vi "uTTA_ucf_WriteChannelCal.vi"(4 "LinGain":dbl, 5 "QuadGain":dbl, 6 "Offset":dbl, 7 "Section":string, 8 "error in (no error)":errorcluster, 9 "Cal Status":T1, 11 "ucf FileRef in":T2) -> (0 "error out":errorcluster, 3 "ucf FileRef out":T2)   [LabVIEW 2021]
uses:
  <vilib>/Utility/config.llb/Config Data RefNum.ctl
  uTTA_Device_Driver/uTTA_Controls/CTL_uTTA_TSP_CalStatus.ctl
  <vilib>/Utility/config.llb/Write Key (U32).vi
  <vilib>/Utility/config.llb/NI_LVConfig.lvlib
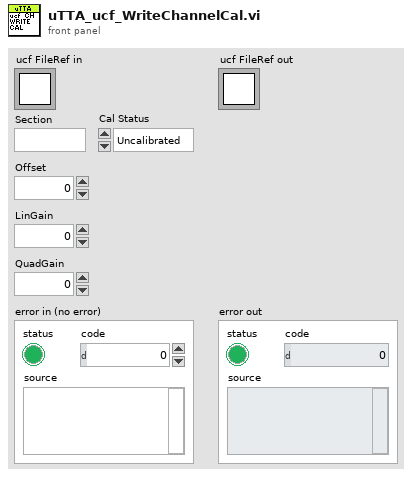
[diagram p1: front panel]
types:
  T1 = typedef "CTL_uTTA_TSP_CalStatus.ctl" = enum16{"Uncalibrated", "Calibrated", "Dummy"}
  T2 = typedef "NI_LVConfig.lvlib/Config Data RefNum.ctl" = refnum<k1>
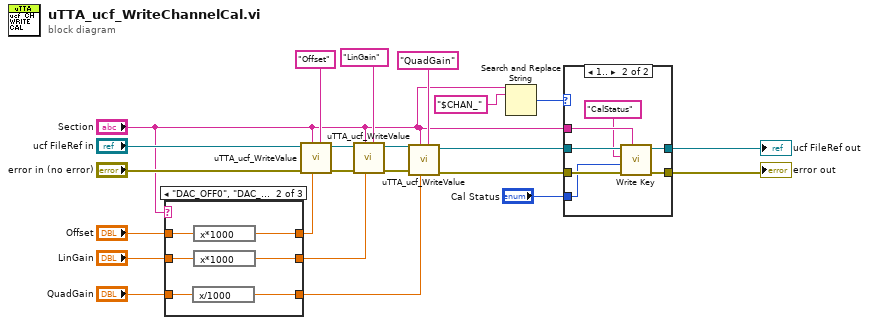
[diagram p0: block diagram]
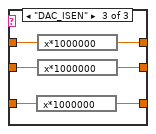
[diagram p4: hidden frame]
diagram:
  n1 = case shown="\"DAC_OFF0\", \"DAC_OFF1\"" "Section" {
    tunnel: "Offset" -> [w26 w30 w36]
    tunnel: "LinGain" -> [w25 w29 w35]
    tunnel: "QuadGain" -> [w24 w32 w38]
    tunnel: [w26 w27 w33] -> w14
    tunnel: [w25 w28 w34] -> w12
    tunnel: [w24 w31 w37] -> w10
    frame Default {
    }
    frame "DAC_OFF0", "DAC_OFF1" {
      n2 = expression code="x/1000"(w32) -> (w31:dbl)
      n3 = expression code="x*1000"(w30) -> (w27:dbl)
      n4 = expression code="x*1000"(w29) -> (w28:dbl)
    }
    frame "DAC_ISEN" {
      n5 = expression code="x*1000000"(w38) -> (w37:dbl)
      n6 = expression code="x*1000000"(w36) -> (w33:dbl)
      n7 = expression code="x*1000000"(w35) -> (w34:dbl)
    }
  }
  n8 = call "uTTA_ucf_WriteValue.vi"("key"="Offset", "Value IN"=w14, "section"="Section", "error in (no error)"="error in (no error)", "ucf-FileRef in"="ucf FileRef in") -> ("error out"=w18:errorcluster, "ucf-FileRef out"=w19:T2)  [unwired: 5 in]
  n9 = call "uTTA_ucf_WriteValue.vi"("key"="LinGain", "Value IN"=w12, "section"="Section", "error in (no error)"=w18, "ucf-FileRef in"=w19) -> ("error out"=w20:errorcluster, "ucf-FileRef out"=w21:T2)  [unwired: 5 in]
  n10 = call "uTTA_ucf_WriteValue.vi"("key"="QuadGain", "Value IN"=w10, "section"="Section", "error in (no error)"=w20, "ucf-FileRef in"=w21) -> ("error out"=w5:errorcluster, "ucf-FileRef out"=w6:T2)  [unwired: 5 in]
  n11 = Search and Replace String(input string="Section", search string="$CHAN_") -> (number of replacements=w7:i32)  [unwired: 6 in, 3 out]
  n12 = case shown="1.." w7 {
    tunnel: w6 -> [w40 w47]
    tunnel: w5 -> [w39 w46]
    tunnel: [w40 w42] -> w3
    tunnel: [w39 w41] -> w4
    tunnel: "Section" -> [_ w44]
    tunnel: "Cal Status" -> [_ w45]
    frame 0, Default {
    }
    frame 1.. {
      n13 = call-poly <vilib>:"Write Key.vi"("section"=w44, "error in (no error)"=w46, "value"=w45, "key"="CalStatus", "refnum"=w47) -> ("error out"=w41:errorcluster, "refnum out"=w42:T2)  [unwired: 4 in, 1 out]
    }
  }
  "ucf FileRef out" <- w3
  "error out" <- w4
